vi "Load Test Sequence (SubVI).vi"(7 "References":T1) -> (15 "Load Test Error":errorcluster)   [LabVIEW 2010]
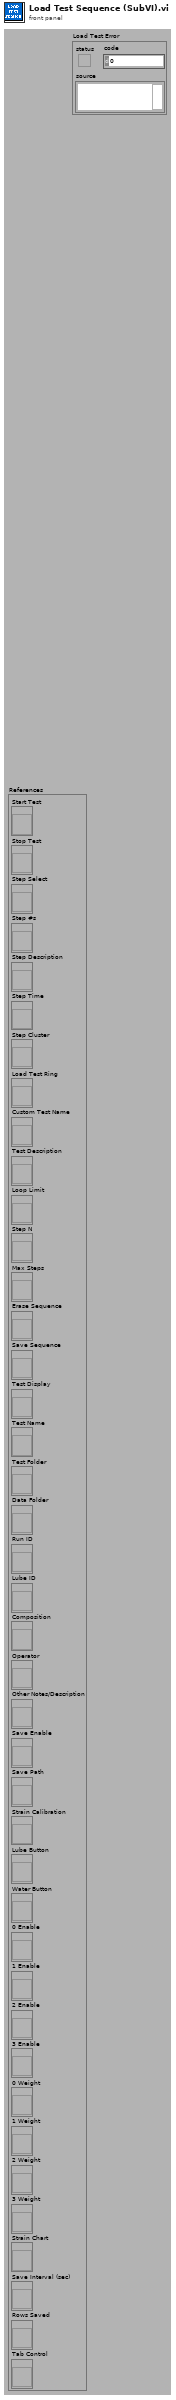
[diagram p1: front panel]
types:
  T1 = cluster{"Start Test":refnum<vi>, "Stop Test":refnum<vi>, "Step Select":refnum<vi>, "Step #s":refnum<vi>, "Step Description":refnum<vi>, "Step Time":refnum<vi>, "Step Cluster":refnum<vi>, "Load Test Ring":refnum<vi>, "Custom Test Name":refnum<vi>, "Test Description":refnum<vi>, "Loop Limit":refnum<vi>, "Step N":refnum<vi>, "Max Steps":refnum<vi>, "Erase Sequence":refnum<vi>, "Save Sequence":refnum<vi>, "Test Display":refnum<vi>, "Test Name":refnum<vi>, "Test Folder":refnum<vi>, "Data Folder":refnum<vi>, "Run ID":refnum<vi>, "Lube ID":refnum<vi>, "Composition":refnum<vi>, "Operator":refnum<vi>, "Other Notes/Description":refnum<vi>, "Save Enable":refnum<vi>, "Save Path":refnum<vi>, "Strain Calibration":refnum<vi>, "Lube Button":refnum<vi>, "Water Button":refnum<vi>, "0 Enable":refnum<vi>, "1 Enable":refnum<vi>, "2 Enable":refnum<vi>, "3 Enable":refnum<vi>, "0 Weight":refnum<vi>, "1 Weight":refnum<vi>, "2 Weight":refnum<vi>, "3 Weight":refnum<vi>, "Strain Chart":refnum<vi>, "Save Interval (sec)":refnum<vi>, "Rows Saved":refnum<vi>, "Tab Control":refnum<vi>}
  T2 = enum8{"Enabled", "Disabled", "Disabled and Grayed Out"}
  T3 = enum16{"open", "replace", "create", "open or create", "replace or create", "replace or create with confirmation"}
  T4 = cluster{"Step Time Unit":u16, "Step End Action":u16, "Relay1":bool, "Relay2":bool}
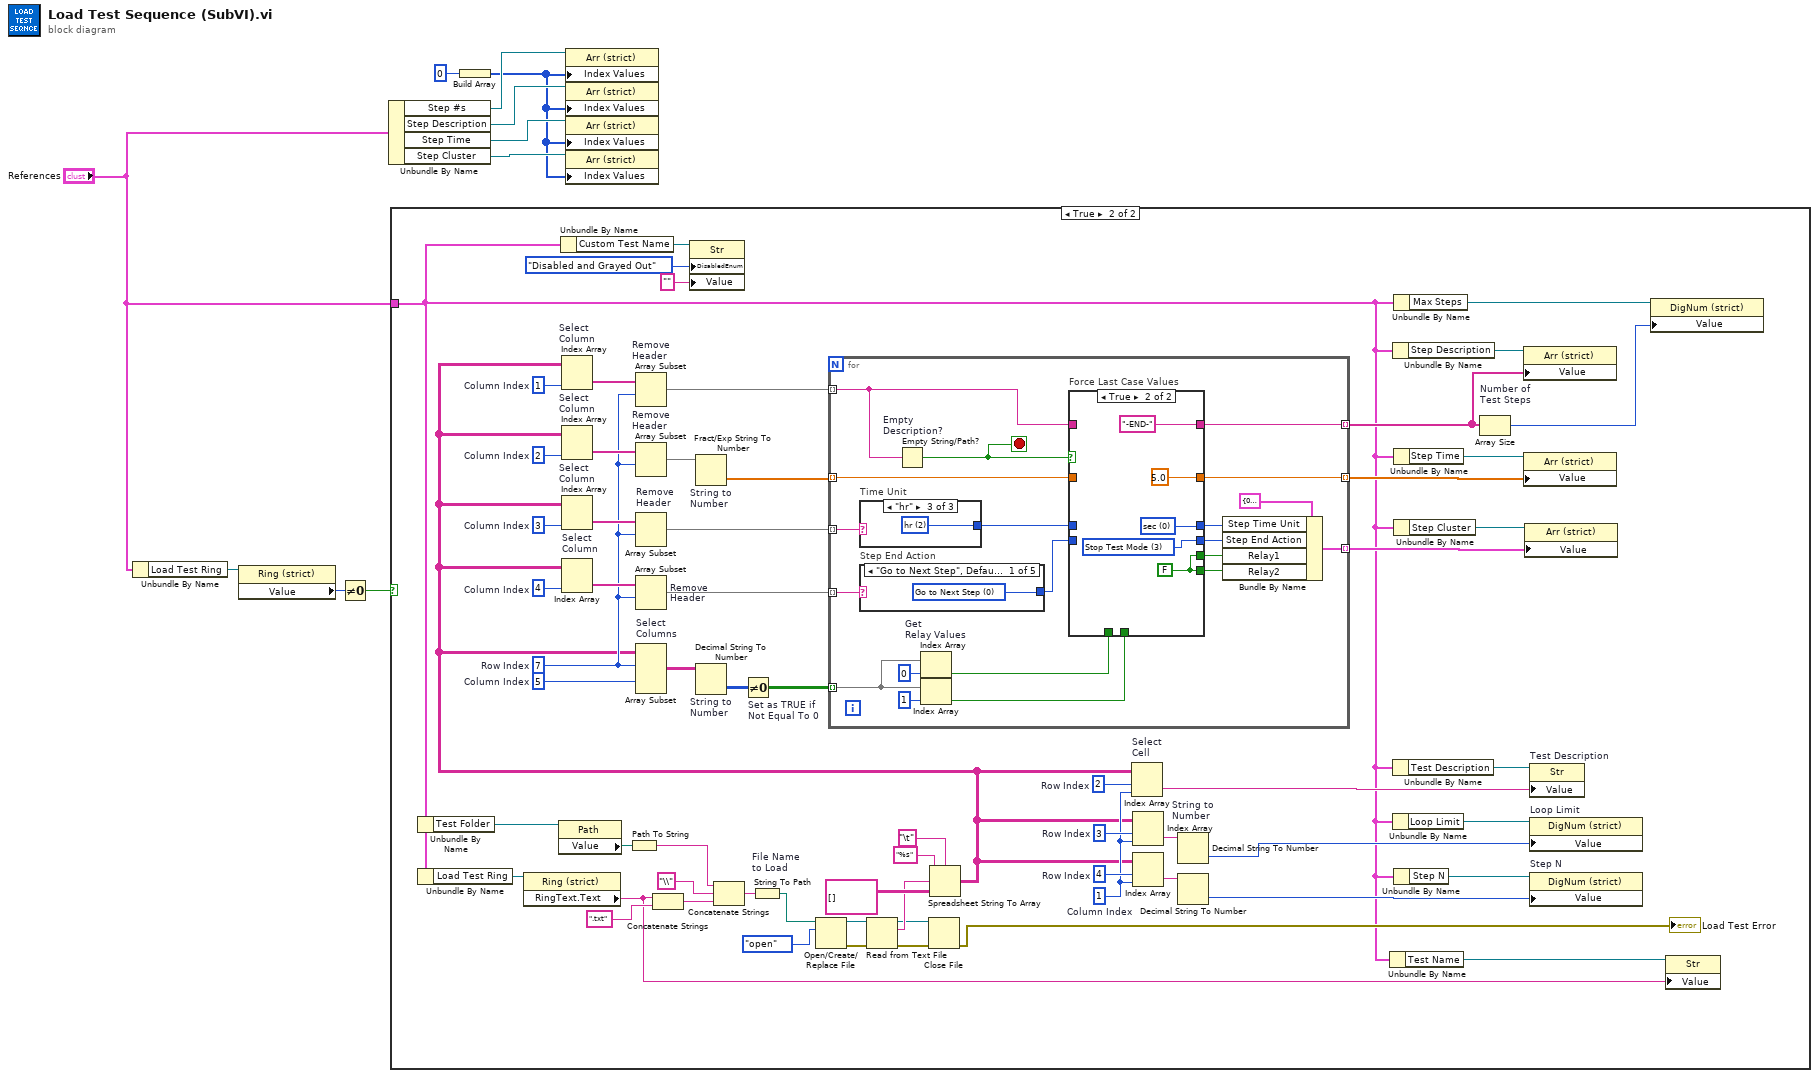
[diagram p0: block diagram]
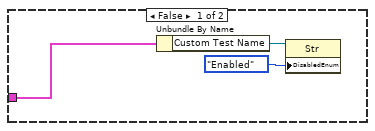
[diagram p2: hidden frame]
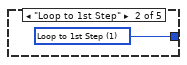
[diagram p4: hidden frame]
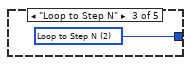
[diagram p5: hidden frame]
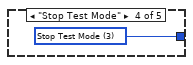
[diagram p6: hidden frame]
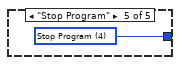
[diagram p7: hidden frame]
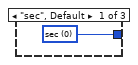
[diagram p8: hidden frame]
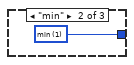
[diagram p9: hidden frame]
diagram:
  n1 = Unbundle By Name("References") -> ("Load Test Ring"=w10:refnum<vi>)
  n2 = property class="Ring (strict)"(reference=w10) -> ("Value"=w9:u16)  [unwired: 1 in, 2 out]
  n3 = Not Equal To 0?(x=w9) -> (x != 0?=w8:bool)
  n4 = Unbundle By Name("References") -> ("Step #s"=w7:refnum<vi>, "Step Description"=w6:refnum<vi>, "Step Time"=w5:refnum<vi>, "Step Cluster"=w4:refnum<vi>)
  n5 = case shown="True" w8 {
    tunnel: "References" -> [w11 w16]
    frame False {
      n6 = Unbundle By Name(w11) -> ("Custom Test Name"=w13:refnum<vi>)
      n7 = property class="Str"(reference=w13, "DisabledEnum"=T2."Enabled" ("Disabled")) -> ()  [unwired: 1 in, 2 out]
    }
    frame True {
      w55 = 2  # Row Index
      w63 = 4  # Row Index
      w65 = 3  # Row Index
      w54 = 1  # Column Index
      w69 = 5  # Column Index
      w70 = 4  # Column Index
      w72 = 3  # Column Index
      w74 = 2  # Column Index
      w68 = 7  # Row Index
      w77 = 1  # Column Index
      n8 = Unbundle By Name(w16) -> ("Test Folder"=w47:refnum<vi>)
      n9 = Unbundle By Name(w16) -> ("Load Test Ring"=w45:refnum<vi>)
      n10 = property class="Ring (strict)"(reference=w45) -> ("RingText.Text"=w19:string)  [unwired: 1 in, 2 out]
      n11 = property class="Path"(reference=w47) -> ("Value"=w46:path)  [unwired: 1 in, 2 out]
      n12 = Unbundle By Name(w16) -> ("Custom Test Name"=w17:refnum<vi>)
      n13 = Path To String(path=w46) -> (string=w56:string)
      n14 = Concatenate Strings(w19, ".txt" ("string")) -> (w43:string)
      n15 = property class="Str"(reference=w17, "DisabledEnum"=T2."Disabled and Grayed Out" ("Disabled"), "Value"="") -> ()  [unwired: 1 in, 2 out]
      n16 = Concatenate Strings(w56, "\\" ("string"), w43) -> (w57:string)
      n17 = String To Path "File Name\nto Load"(string=w57) -> (path=w26:path)
      n18 = Open/Create/Replace File(file path (use dialog)=w26, operation (0:open)=T3."open") -> (refnum out=w22:refnum<file>, error out=w31:errorcluster)  [unwired: 4 in, 1 out]
      n19 = Read from Text File(file (use dialog)=w22, error in=w31) -> (refnum out=w21:refnum<file>, text=w25:string, error out=w32:errorcluster)  [unwired: 3 out]
      n20 = Close File(refnum=w21, error in=w32) -> (error out=→"Load Test Error":errorcluster)  [unwired: 1 out]
      n21 = Spreadsheet String To Array(delimiter (Tab)="\t" ("delimiter (\\t)"), format string="%s" ("format (%s)"), spreadsheet string=w25, array type (2D Dbl)=string[][] [] ("appended array")) -> (array=w24:string[][])
      n22 = Index Array "Select\nColumn"(array=w24, index (col)=w77) -> (element=w76:string[])  [unwired: 1 in]
      n23 = Index Array "Select\nColumn"(array=w24, index (col)=w74) -> (element=w75:string[])  [unwired: 1 in]
      n24 = Index Array "Select\nColumn"(array=w24, index (col)=w72) -> (element=w73:string[])  [unwired: 1 in]
      n25 = Index Array "Select\nColumn"(array=w24, index (col)=w70) -> (element=w71:string[])  [unwired: 1 in]
      n26 = Array Subset "Remove\nHeader"(array=w76, index=w68) -> (w51:string[])  [unwired: 1 in]
      n27 = Array Subset "Remove\nHeader"(array=w75, index=w68) -> (w59:string[])  [unwired: 1 in]
      n28 = Array Subset "Remove\nHeader"(array=w73, index=w68) -> (w49:string[])  [unwired: 1 in]
      n29 = Array Subset "Remove\nHeader"(array=w71, index=w68) -> (w48:string[])  [unwired: 1 in]
      n30 = Array Subset "Select\nColumns"(array=w24, index (row)=w68, index (col)=w69) -> (w67:string[][])  [unwired: 2 in]
      n31 = Fract/Exp String To Number "String to\nNumber"(string=w59) -> (number=w50:dbl[])  [unwired: 3 in, 1 out]
      n32 = Decimal String To Number "String to\nNumber"(string=w67) -> (number=w66:i32[][])  [unwired: 2 in, 1 out]
      n33 = Not Equal To 0? "Set as TRUE if\nNot Equal To 0"(x=w66) -> (x != 0?=w52:bool[][])
      n34 = for {
        tunnel: w51 -> [w79] mode=indexing
        tunnel: [w78] -> w37 mode=indexing
        tunnel: w52 -> [w97] mode=indexing
        tunnel: w50 -> [w91] mode=indexing
        tunnel: w49 -> [w96] mode=indexing
        tunnel: w48 -> [w95] mode=indexing
        tunnel: [w90] -> w39 mode=indexing
        tunnel: [w80] -> w42 mode=indexing
        stop <- w81 stop-if-true
        n35 = case "Time Unit" shown="\"hr\"" w96 {
          tunnel: [w114 w115 w116] -> w88
          frame "sec", Default {
            w114 = u16 0 items=["sec", "min", "hr"] ("Step Time Unit")
          }
          frame "min" {
            w115 = u16 1 items=["sec", "min", "hr"] ("Step Time Unit")
          }
          frame "hr" {
            w116 = u16 2 items=["sec", "min", "hr"] ("Step Time Unit")
          }
        }
        n36 = case "Step End Action" shown="\"Go to Next Step\", Default" w95 {
          tunnel: [w109 w110 w111 w112 w113] -> w87
          frame "Go to Next Step", Default {
            w109 = u16 0 items=["Go to Next Step", "Loop to 1st Step", "Loop to Step N", "Stop Test Mode", "Stop Program"] ("Step End Action")
          }
          frame "Loop to 1st Step" {
            w110 = u16 1 items=["Go to Next Step", "Loop to 1st Step", "Loop to Step N", "Stop Test Mode", "Stop Program"] ("Step End Action")
          }
          frame "Loop to Step N" {
            w111 = u16 2 items=["Go to Next Step", "Loop to 1st Step", "Loop to Step N", "Stop Test Mode", "Stop Program"] ("Step End Action")
          }
          frame "Stop Test Mode" {
            w112 = u16 3 items=["Go to Next Step", "Loop to 1st Step", "Loop to Step N", "Stop Test Mode", "Stop Program"] ("Step End Action")
          }
          frame "Stop Program" {
            w113 = u16 4 items=["Go to Next Step", "Loop to 1st Step", "Loop to Step N", "Stop Test Mode", "Stop Program"] ("Step End Action")
          }
        }
        n37 = Empty String/Path? "Empty\nDescription?"(string/path=w79) -> (empty?=w81:bool)
        n38 = Index Array "Get\nRelay Values"(array=w97, index=0) -> (element=w83:bool)
        n39 = Index Array(array=w97, index=1) -> (element=w82:bool)
        n40 = case "Force Last Case Values" shown="True" w81 {
          tunnel: w91 -> [w103 _]
          tunnel: [w103 5.0] -> w90
          tunnel: [w102 w107] -> w89
          tunnel: w88 -> [w102 _]
          tunnel: w87 -> [w101 _]
          tunnel: [w101 w106] -> w86
          tunnel: [w99 w105] -> w85
          tunnel: [w100 w105] -> w84
          tunnel: w83 -> [w100 _]
          tunnel: w82 -> [w99 _]
          tunnel: w79 -> [w98 _]
          tunnel: [w98 "-END-"] -> w78
          frame False {
          }
          frame True {
            w105 = FALSE
            w106 = u16 3 items=["Go to Next Step", "Loop to 1st Step", "Loop to Step N", "Stop Test Mode", "Stop Program"] ("Step End Action")
            w107 = u16 0 items=["sec", "min", "hr"] ("Step Time Unit")
          }
        }
        n41 = Bundle By Name(cluster=T4 {"Step Time Unit"=0, "Step End Action"=0, "Relay1"=FALSE, "Relay2"=FALSE} ("Step Cluster"), "Step Time Unit"=w89, "Step End Action"=w86, "Relay1"=w84, "Relay2"=w85) -> (w80:T4)
      }
      n42 = Index Array "Select\nCell"(array=w24, index (row)=w55, index (col)=w54) -> (element=w53:string)
      n43 = Index Array(array=w24, index (row)=w65, index (col)=w54) -> (element=w62:string)
      n44 = Index Array(array=w24, index (row)=w63, index (col)=w54) -> (element=w64:string)
      n45 = Decimal String To Number "String to\nNumber"(string=w62) -> (number=w60:i32)  [unwired: 2 in, 1 out]
      n46 = Decimal String To Number(string=w64) -> (number=w61:i32)  [unwired: 2 in, 1 out]
      n47 = Unbundle By Name(w16) -> ("Test Name"=w20:refnum<vi>)
      n48 = Unbundle By Name(w16) -> ("Step Description"=w38:refnum<vi>)
      n49 = Unbundle By Name(w16) -> ("Test Description"=w36:refnum<vi>)
      n50 = Unbundle By Name(w16) -> ("Loop Limit"=w35:refnum<vi>)
      n51 = Unbundle By Name(w16) -> ("Max Steps"=w33:refnum<vi>)
      n52 = Unbundle By Name(w16) -> ("Step Time"=w40:refnum<vi>)
      n53 = Unbundle By Name(w16) -> ("Step Cluster"=w41:refnum<vi>)
      n54 = Unbundle By Name(w16) -> ("Step N"=w34:refnum<vi>)
      n55 = Array Size "Number of\nTest Steps"(array=w37) -> (size(s)=w14:i32)
      n56 = property class="Arr (strict)"(reference=w38, "Value"=w37) -> ()  [unwired: 1 in, 2 out]
      n57 = property class="Arr (strict)"(reference=w40, "Value"=w39) -> ()  [unwired: 1 in, 2 out]
      n58 = property class="Arr (strict)"(reference=w41, "Value"=w42) -> ()  [unwired: 1 in, 2 out]
      n59 = property on="Test Description" class="Str"(reference=w36, "Value"=w53) -> ()  [unwired: 1 in, 2 out]
      n60 = property on="Loop Limit" class="DigNum (strict)"(reference=w35, "Value"=w60) -> ()  [unwired: 1 in, 2 out]
      n61 = property on="Step N" class="DigNum (strict)"(reference=w34, "Value"=w61) -> ()  [unwired: 1 in, 2 out]
      n62 = property class="DigNum (strict)"(reference=w33, "Value"=w14) -> ()  [unwired: 1 in, 2 out]
      n63 = property class="Str"(reference=w20, "Value"=w19) -> ()  [unwired: 1 in, 2 out]
    }
  }
  n64 = Build Array(u32 0) -> (w3:u32[])
  n65 = property class="Arr (strict)"(reference=w7, "Index Values"=w3) -> ()  [unwired: 1 in, 2 out]
  n66 = property class="Arr (strict)"(reference=w6, "Index Values"=w3) -> ()  [unwired: 1 in, 2 out]
  n67 = property class="Arr (strict)"(reference=w5, "Index Values"=w3) -> ()  [unwired: 1 in, 2 out]
  n68 = property class="Arr (strict)"(reference=w4, "Index Values"=w3) -> ()  [unwired: 1 in, 2 out]
